vi "Polymorphic - Send Initialization Command to DAQ.vi"   [LabVIEW 2021]
doc: "Send a series of commands to initialize the DAQ device.\nTurn echo on, stop any data streaming, set power state, set data format to JSON."
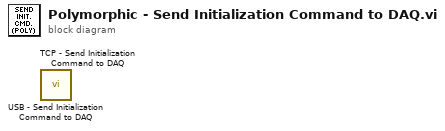
[diagram p0: block diagram]
diagram:
  n1 = call "USB - Send Initialization Command to DAQ.vi"() -> ()  [unwired: 10 in, 2 out]
  n2 = call "TCP - Send Initialization Command to DAQ.vi"() -> ()  [unwired: 10 in, 2 out]
